vi "Visa_Serial_Port_Init.vi"(1 "flow control etc.":T1={"input XON/XOFF"=FALSE, "input HW Handshake"=FALSE, "input alt HW HShk"=FALSE, "output XON/XOFF"=FALSE, "output HW Handshake"=FALSE, "output alt HW HShk"=FALSE, "XOFF byte "=19, "XON byte"=17, "parity error byte"=0} {"parity error byte" format="%x"; "XON byte" format="%x"; "XOFF byte" format="%x"}, 2 "parity":T2(ring), 3 "buffer size":u16, 4 "stop bits":enum16{"1 bit", "1.5 bits", "2 bits"}(ring), 5 "data bits":u16=8 min=5 max=8 step=1, 6 "baud rate":u32=9600, 7 "Visa Port Name":refnum<visa-resource-name>) -> (0 "error out":errorcluster)   [LabVIEW 2010]
doc: "Initializes the selected serial port to the specified settings.\n\n<B>Note</B> This VI might clear the buffer of any existing data. You should use this VI only if you want to reset the serial port completely.\n\n<B>Note:</B> This VI was removed from the Functions palette. Use the VIs and functions on the VISA palette to control serial devices. If you use the LabVIEW PDA Module, use this VI for serial communication."
uses:
  <vilib>/Instr/_visa.llb/VISA Configure Serial Port (Instr).vi
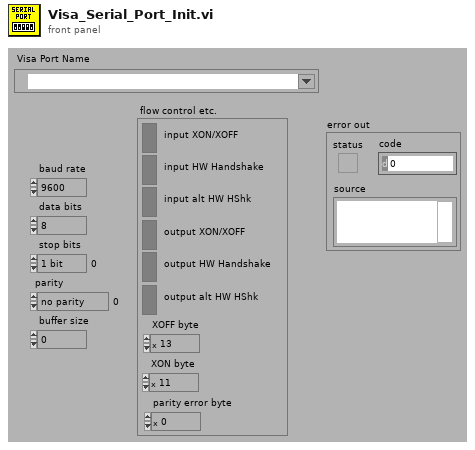
[diagram p1: front panel]
types:
  T1 = cluster{"input XON/XOFF":bool, "input HW Handshake":bool, "input alt HW HShk":bool, "output XON/XOFF":bool, "output HW Handshake":bool, "output alt HW HShk":bool, "XOFF byte ":u8, "XON byte":u8, "parity error byte":u16}
  T2 = enum16{"no parity", "odd parity", "even parity", "mark parity", "space parity"}
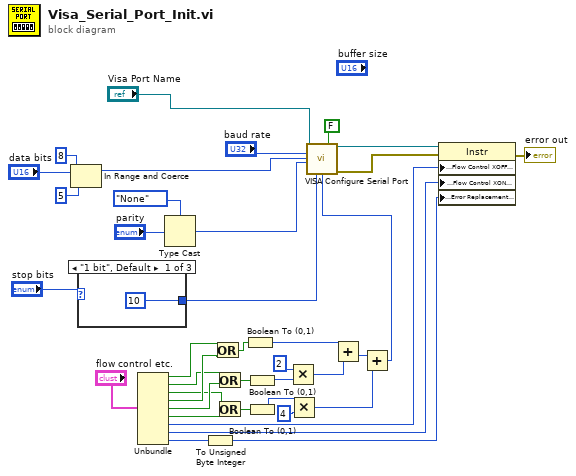
[diagram p0: block diagram]
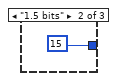
[diagram p2: hidden frame]
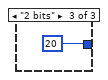
[diagram p3: hidden frame]
diagram:
  n1 = In Range and Coerce(upper limit=u16 8, x="data bits", lower limit=u16 5) -> (coerced(x)=w35:u16)  [unwired: 1 out]
  n2 = case shown="\"1 bit\", Default" "stop bits" {
    tunnel: [u16 10 u16 15 u16 20] -> w30
    frame "1 bit", Default {
    }
    frame "1.5 bits" {
    }
    frame "2 bits" {
    }
  }
  n3 = Unbundle("flow control etc.") -> ("input XON/XOFF"=w24:bool, "input HW Handshake"=w21:bool, "input alt HW HShk"=w19:bool, "output XON/XOFF"=w23:bool, "output HW Handshake"=w20:bool, "output alt HW HShk"=w18:bool, "XOFF byte"=w28:u8, "XON byte"=w27:u8, "parity error byte"=w26:u16)
  n4 = Type Cast(type=enum16{"None", "Odd", "Even", "Mark", "Space"}."None" ("parity (0:none)"), x="parity") -> (*(type *) &x=w32:enum16{"None", "Odd", "Even", "Mark", "Space"})
  n5 = To Unsigned Byte Integer(number=w26) -> (unsigned 8bit integer=w25:u8)
  n6 = Or(x=w24, y=w23) -> (x .or. y?=w22:bool)
  n7 = Or(x=w21, y=w20) -> (x .or. y?=w17:bool)
  n8 = Or(x=w19, y=w18) -> (x .or. y?=w16:bool)
  n9 = Boolean To (0,1)(Boolean=w22) -> (0, 1=w11:i16)
  n10 = Boolean To (0,1)(Boolean=w17) -> (0, 1=w14:i16)
  n11 = Boolean To (0,1)(Boolean=w16) -> (0, 1=w12:i16)
  n12 = Multiply(x=u16 2 ("y"), y=w14) -> (x*y=w10:u16)
  n13 = Multiply(x=w12, y=u16 4) -> (x*y=w9:u16)
  n14 = Add(x=w11, y=w10) -> (x+y=w8:u16)
  n15 = Add(x=w8, y=w9) -> (x+y=w7:u16)
  n16 = call-poly "VISA Configure Serial Port"("VISA resource name"="Visa Port Name", "Enable Termination\nChar (T)"=FALSE ("Enable Termination\nChar (T)"), "baud rate (9600)"="baud rate", "data bits (8)"=w35, "parity (0:none)"=w32, "stop bits (10: 1 bit)"=w30, "flow control (0:none)"=w7) -> ("VISA resource name out"=w4:refnum<visa-resource-name>, "error out"=w3:errorcluster)  [unwired: 1 in, 6 out]
  n17 = property class="Instr"(reference=w4, error in=w3, "Serial Settings:Flow Control XOFF Character"=w28, "Serial Settings:Flow Control XON Character"=w27, "Serial Settings:Error Replacement Character"=w25) -> (error out=→"error out":errorcluster)  [unwired: 1 out]
